vi "VCS Activate Position Compare.vi"(8 "error in (no error)":errorcluster, 9 "polarity":i32, 10 "digitalOutputNumber":u16, 11 "axis in":cluster{"keyHandle":u32, "nodeId":u16}={"keyHandle"=0, "nodeId"=1}) -> (0 "error out":errorcluster, 3 "axis out":cluster{"keyHandle":u32, "nodeId":u16}={"keyHandle"=0, "nodeId"=1})   [LabVIEW 2019, in "maxonEPOS.lvlib"]
doc: "<B>VCS_ActivatePositionCompare</B> enables the output to position compare method."
uses:
  Examples/maxonEPOS.lvlib
  Resources/EposCmd.dll
  Resources/EposCmd64.dll
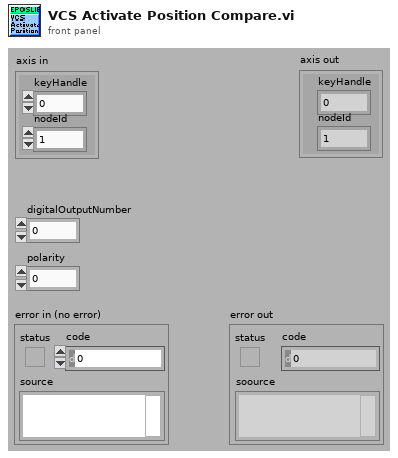
[diagram p1: front panel]
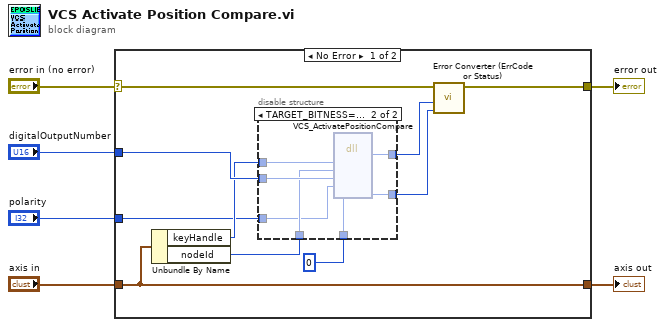
[diagram p0: block diagram]
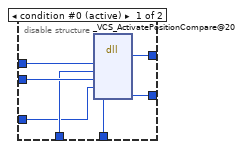
[diagram p2: hidden frame]
diagram:
  n1 = case shown="No Error" "error in (no error)" {
    selector: "error in (no error)" -> [w14 w31]
    tunnel: "axis in" -> [w16 w32]
    tunnel: [w16 w32] -> w5
    tunnel: [w15 w31] -> w4
    tunnel: "digitalOutputNumber" -> [w12 _]
    tunnel: "polarity" -> [w7 _]
    frame No Error {
      n2 = Unbundle By Name(w16) -> ("keyHandle"=w10:u32, "nodeId"=w11:u16)
      n3 = disable-structure shown="TARGET_BITNESS==64" {
        disable-tunnel: u32 0 ("pErrorCode") -> [w23 w30]
        disable-tunnel: w12 -> [w22 w29]
        disable-tunnel: w11 -> [w21 w28]
        disable-tunnel: w10 -> [w20 w27]
        disable-tunnel: [w19 w26] -> w9
        disable-tunnel: [w18 w25] -> w8
        disable-tunnel: w7 -> [w17 w24]
        frame condition #0 (active) {
          n4 = dll-call lib="C:/workspace/project/scancon/sw/SSI_Tool/InstrumentsInterfaces/Motordriver/maxon EPOS/Resources/EposCmd.*" fn="_VCS_ActivatePositionCompare@20"("KeyHandle"=w20, "NodeId"=w21, "DigitalOutputNumber"=w22, "Polarity"=w17, "pErrorCode"=w23) -> (w19:i32, "pErrorCode"=w18:u32)  [unwired: 7 in, 2 out]
        }
        frame condition #1 {
          n5 = dll-call lib="C:/setup/Resources/EposCmd64.*" fn="VCS_ActivatePositionCompare" ("EposCmd.dll:_VCS_ActivatePositionCompare@20")("KeyHandle"=w27, "NodeId"=w28, "DigitalOutputNumber"=w29, "Polarity"=w24, "pErrorCode"=w30) -> ("Rückgabetyp"=w26:i32, "pErrorCode"=w25:u32)  [unwired: 7 in, 2 out]
        }
      }
      n6 = call "Error Converter (ErrCode or Status).vi"("error code"=w8, "return type"=w9, "error in (no error)"=w14) -> ("error out"=w15:errorcluster)  [unwired: 7 in]
    }
    frame Error {
    }
  }
  "error out" <- w4
  "axis out" <- w5
